vi "Backup File or Folder.vi"(8 "error in (no error)":errorcluster, 11 "File/Directory Path":path) -> (0 "error out":errorcluster, 3 "File/Directory Path (dup)":path)   [LabVIEW 2019]
doc: "Backup the file at the provided location (by creating a copy with ~added in front of the file name) and returns the original path for deletion (or other use).\nIf the file doesn't exist, returns an error."
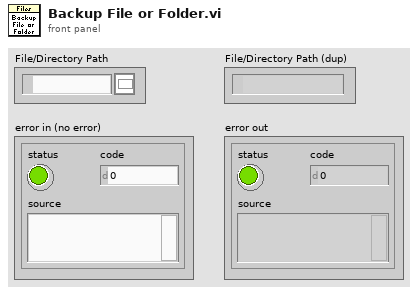
[diagram p1: front panel]
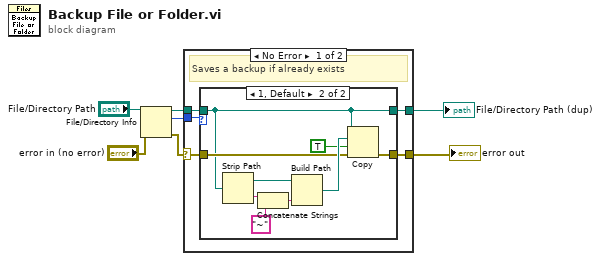
[diagram p0: block diagram]
diagram:
  n1 = File/Directory Info(path="File/Directory Path", error in="error in (no error)") -> (path out=w4:path, size=w2:i64, error out=w1:errorcluster)  [unwired: 4 out]
  n2 = case shown="No Error" w1 {
    selector: w1 -> [w10 w24]
    tunnel: w4 -> [w11 w25]
    tunnel: [w12 w24] -> w5
    tunnel: [w8 w25] -> w7
    tunnel: w2 -> [w9 _]
    frame No Error {
      # "Saves a backup if already exists"
      n3 = case shown="1, Default" w9 {
        tunnel: [w14 w17] -> w12
        tunnel: w11 -> [w13 w15]
        tunnel: w10 -> [w14 w16]
        tunnel: [w13 w15] -> w8
        frame 0 {
        }
        frame 1, Default {
          n4 = Strip Path(path=w15) -> (stripped path=w23:path, name=w22:string)
          n5 = Concatenate Strings(w22, "~" ("string")) -> (w21:string)
          n6 = Build Path(base path=w23, name or relative path=w21) -> (appended path=w19:path)
          n7 = Copy(8:w16, 9:TRUE ("overwrite (F)"), 10:w19, 11:w15) -> (0:w17:errorcluster)  [unwired: 1 in, 2 out]
        }
      }
    }
    frame Error {
      # "File does not exist, etc.: create later"
    }
  }
  "File/Directory Path (dup)" <- w7
  "error out" <- w5
